vi "lfieldpanel_generate_user_events.vi"(8 "error in (no error)":errorcluster, 11 "lightfield_panel in":refnum<class "lightfield_panel.lvclass">) -> (0 "error out":errorcluster, 2 "lfield_ui_events":T1, 3 "lightfield_panel out":refnum<class "lightfield_panel.lvclass">)   [LabVIEW 2015, in "lightfield_panel.lvclass"]
uses:
  lightfield_panel.lvclass
  lfield_ui_event_refs.ctl
  lfield_ui_events.ctl
  lightfield_panel.lvclass/lightfield_panel.ctl
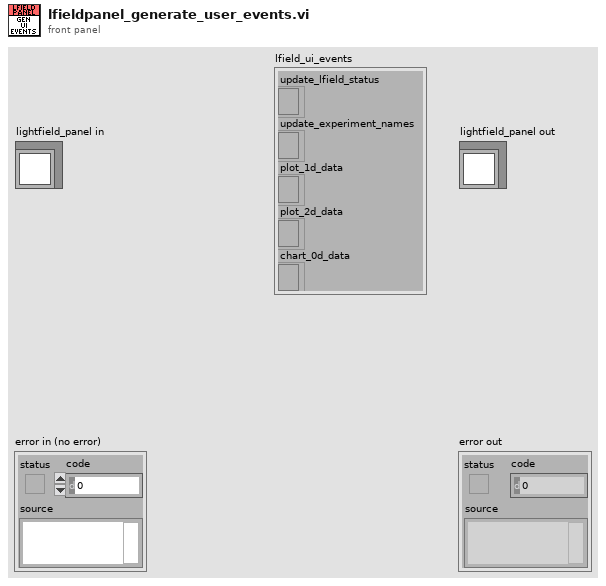
[diagram p1: front panel]
types:
  T1 = typedef "lfield_ui_event_refs.ctl" = cluster{"update_lfield_status":refnum<event-registration>, "update_experiment_names":refnum<event-registration>, "plot_1d_data":refnum<event-registration>, "plot_2d_data":refnum<event-registration>, "chart_0d_data":refnum<event-registration>}
  T2 = typedef "lfield_ui_events.ctl" = cluster{"update_lfield_status":refnum<user-event>, "update_experiment_names":refnum<user-event>, "plot_1d_data":refnum<user-event>, "plot_2d_data":refnum<user-event>, "chart_0d_data":refnum<user-event>}
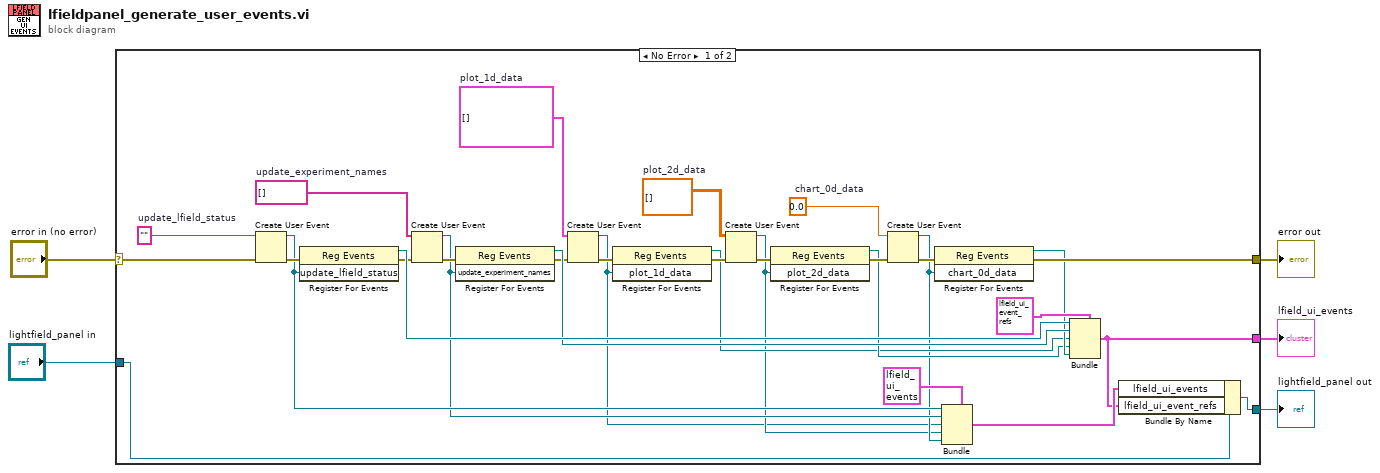
[diagram p0: block diagram]
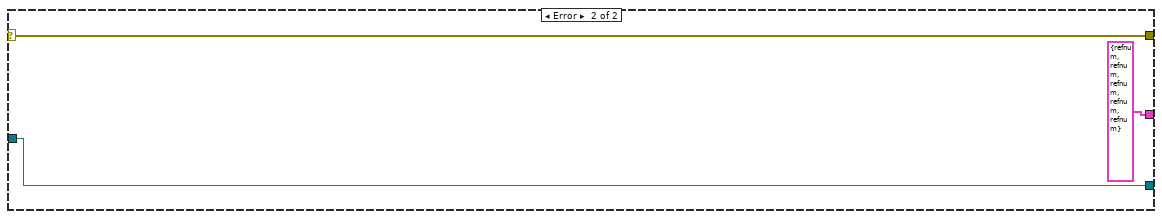
[diagram p2: hidden frame]
diagram:
  n1 = case shown="No Error" "error in (no error)" {
    selector: "error in (no error)" -> [w33 w40]
    tunnel: [w13 w40] -> w3
    tunnel: [w37 w39] -> w2
    tunnel: "lightfield_panel in" -> [w32 w39]
    tunnel: [w27 T1 {"update_lfield_status"=refnum, "update_experiment_names"=refnum, "plot_1d_data"=refnum, "plot_2d_data"=refnum, "chart_0d_data"=refnum} ("output cluster")] -> w1
    frame No Error {
      w16 = 0.0  # chart_0d_data
      w18 = dbl[][] []  # plot_2d_data
      w19 = cluster{dbl[], dbl[]}[] []  # plot_1d_data
      w24 = string[] []  # update_experiment_names
      w36 = ""  # update_lfield_status
      n2 = Create User Event(user event datatype=w36, error in=w33) -> (user event=w31:refnum<user-event>, error out=w35:errorcluster)
      n3 = register-events(error in=w35, w31) -> (reference out=w34:refnum<event-registration>, error out=w26:errorcluster)  [unwired: 1 in]
      n4 = Create User Event(user event datatype=w24, error in=w26) -> (user event=w22:refnum<user-event>, error out=w25:errorcluster)
      n5 = register-events(error in=w25, w22) -> (reference out=w23:refnum<event-registration>, error out=w14:errorcluster)  [unwired: 1 in]
      n6 = Create User Event(user event datatype=w19, error in=w14) -> (user event=w6:refnum<user-event>, error out=w21:errorcluster)
      n7 = register-events(error in=w21, w6) -> (reference out=w9:refnum<event-registration>, error out=w12:errorcluster)  [unwired: 1 in]
      n8 = Create User Event(user event datatype=w18, error in=w12) -> (user event=w7:refnum<user-event>, error out=w20:errorcluster)
      n9 = register-events(error in=w20, w7) -> (reference out=w10:refnum<event-registration>, error out=w15:errorcluster)  [unwired: 1 in]
      n10 = Create User Event(user event datatype=w16, error in=w15) -> (user event=w8:refnum<user-event>, error out=w17:errorcluster)
      n11 = register-events(error in=w17, w8) -> (reference out=w11:refnum<event-registration>, error out=w13:errorcluster)  [unwired: 1 in]
      n12 = Bundle(cluster=T2 {"update_lfield_status"=refnum, "update_experiment_names"=refnum, "plot_1d_data"=refnum, "plot_2d_data"=refnum, "chart_0d_data"=refnum} ("output cluster"), "update_lfield_status"=w31, "update_experiment_names"=w22, "plot_1d_data"=w6, "plot_2d_data"=w7, "chart_0d_data"=w8) -> (w29:T2)
      n13 = Bundle(cluster=T1 {"update_lfield_status"=refnum, "update_experiment_names"=refnum, "plot_1d_data"=refnum, "plot_2d_data"=refnum, "chart_0d_data"=refnum} ("output cluster"), "update_lfield_status"=w34, "update_experiment_names"=w23, "plot_1d_data"=w9, "plot_2d_data"=w10, "chart_0d_data"=w11) -> (w27:T1)
      n14 = Bundle By Name(cluster=w32, "lfield_ui_events"=w29, "lfield_ui_event_refs"=w27) -> (w37:refnum<class "lightfield_panel.lvclass">)
    }
    frame Error {
    }
  }
  "error out" <- w3
  "lightfield_panel out" <- w2
  "lfield_ui_events" <- w1
